vi "Test - Inversor - Request Simple 1.vi"(8 "error in":errorcluster, 11 "Module ID":i32) -> (0 "error out":errorcluster, 3 "Pass":bool)   [LabVIEW 2019]
doc: "_____\nCreated using DQMH Framework: Event Scripter 7.1.0.1503."
uses:
  Libraries/Inversor/Inversor.lvlib
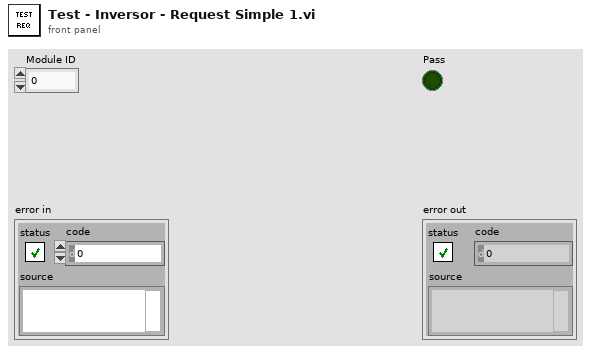
[diagram p1: front panel]
types:
  T1 = typedef "Inversor.lvlib/Broadcast Events--cluster.ctl" = cluster{"Module Did Init":refnum<user-event>, "Status Updated":refnum<user-event>, "Error Reported":refnum<user-event>, "Module Did Stop":refnum<user-event>, "Update Module Execution Status":refnum<user-event>}
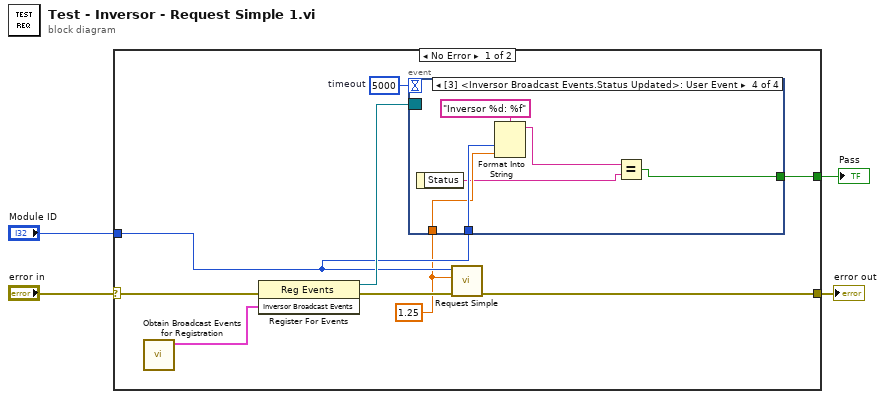
[diagram p0: block diagram]
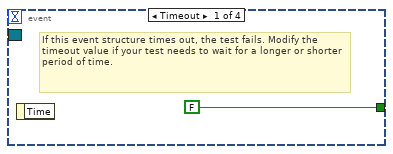
[diagram p2: hidden frame]
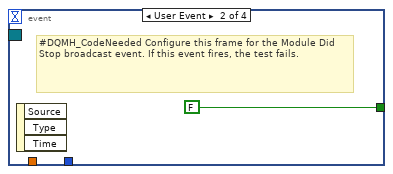
[diagram p3: hidden frame]
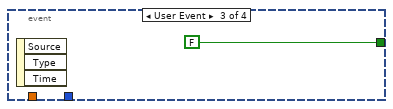
[diagram p4: hidden frame]
diagram:
  n1 = case shown="No Error" "error in" {
    selector: "error in" -> [w13 w23]
    tunnel: [w12 w23] -> w3
    tunnel: "Module ID" -> [w6 _]
    tunnel: [w7 _] -> w1
    frame No Error {
      w5 = 1.25 ("Numeric")
      w8 = 5000  # timeout
      n2 = call "Obtain Broadcast Events for Registration.vi"() -> ("Inversor Broadcast Events"=w10:T1)  [unwired: 9 in, 2 out]
      n3 = register-events(error in=w13, w10) -> (reference out=w9:refnum<event-registration>, error out=w11:errorcluster)  [unwired: 1 in]
      n4 = event shown="[3] <Inversor Broadcast Events.Status Updated>: User Event" {
        selector: w9 -> [_ _ _ _]
        dyn-events: _ -> [_ _ _ _]
        timeout: w8 -> [_ _ _ _]
        tunnel: [FALSE FALSE FALSE w18] -> w7
        tunnel: w6 -> [_ _ _ w22]
        tunnel: w5 -> [_ _ _ w21]
        event Timeout {
          # "If this event structure times out, the test fails. Modify the timeout value if your test needs to wait for a longer or shorter period of time."
          n5 = event-data() -> ()  [unwired: 1 in, 1 out]
        }
        event User Event {
          # "#DQMH_CodeNeeded Configure this frame for the Module Did Stop broadcast event. If this event fires, the test fails."
          n6 = event-data() -> ()  [unwired: 1 in, 3 out]
        }
        event User Event {
          n7 = event-data() -> ()  [unwired: 1 in, 3 out]
        }
        event User Event {
          n8 = event-data() -> ("Status"=w19:string)  [unwired: 1 in]
          n9 = Format Into String(format string="Inversor %d: %f", w22, w21) -> (resulting string=w20:string)  [unwired: 2 in, 1 out]
          n10 = Equal?(x=w20, y=w19) -> (x = y?=w18:bool)
        }
      }
      n11 = call "Request Simple.vi"("error in"=w11, "Numeric"=w5, "Module ID"=w6) -> ("error out"=w12:errorcluster)  [unwired: 8 in]
    }
    frame Error {
    }
  }
  "error out" <- w3
  "Pass" <- w1
